vi "tokenizer.vi"(11 "Input String":string) -> (1 "timestamp":string, 2 "room":string, 3 "mote data":string)   [LabVIEW 2011]
panel:
  out "output string":string
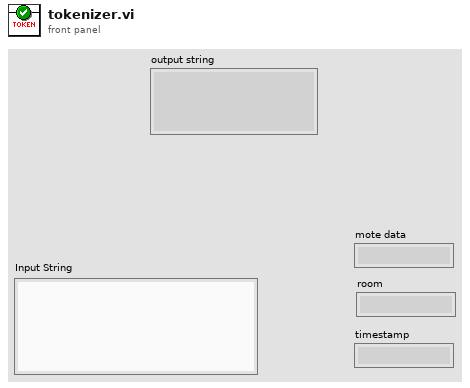
[diagram p1: front panel]
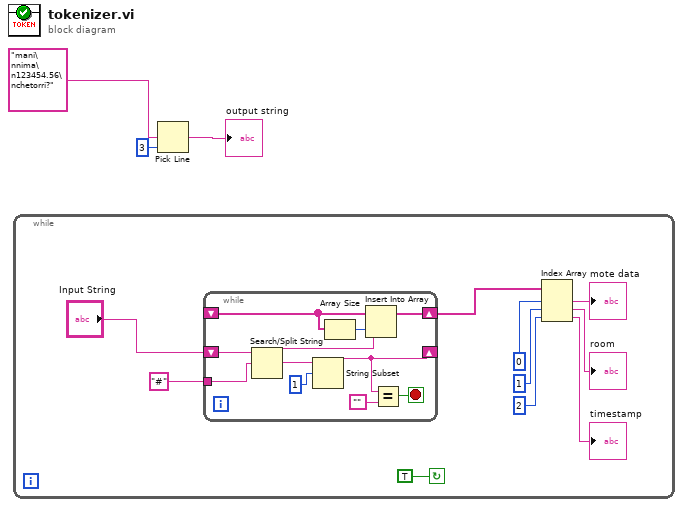
[diagram p0: block diagram]
diagram:
  n1 = while {
    stop <- TRUE continue-if-true
    n2 = while {
      shift-right: [w15] -> _
      shift-left: "Input String" -> [w24]
      shift-right: [w17] -> w5
      shift-left: _ -> [w19]
      tunnel: "#" ("search string/char (-)") -> [w14]
      stop <- w16 stop-if-true
      n3 = Search/Split String(string=w24, search string/char (-)=w14) -> (substring before match=w21:string, match + rest of string=w23:string)  [unwired: 1 in, 1 out]
      n4 = String Subset(string=w23, offset (0)=1) -> (substring=w15:string)  [unwired: 1 in]
      n5 = Array Size(array=w19) -> (size(s)=w20:i32)
      n6 = Insert Into Array(array=w19, index=w20, new element=w21) -> (w17:string[])
      n7 = Equal?(x=w15, y="") -> (x = y?=w16:bool)
    }
    n8 = Index Array(array=w5, index #1=0 ("index"), index #2=1 ("index"), index #3=2 ("index")) -> (element #1=→"mote data":string, element #2=→"room":string, element #3=→"timestamp":string)
  }
  n9 = Pick Line(multi-line string="mani\nnima\n123454.56\nchetorri?", line index=3) -> (output string=→"output string":string)  [unwired: 1 in]
